vi "Check Axis Faults.vi"(8 "error in (no error)":errorcluster, 11 "Gantry in":refnum<class "Gantry.lvclass">) -> (0 "error out":errorcluster, 3 "Gantry out":refnum<class "Gantry.lvclass">)   [LabVIEW 2026, in "Gantry.lvclass"]
uses:
  Gantry.lvclass
  <instrlib>/Aerotech Automation1/Status/TypeDefs/Axis Fault Cluster.ctl
  <instrlib>/Aerotech Automation1/Status/TypeDefs/Axis Status Items Cluster.ctl
  <instrlib>/Aerotech Automation1/Status/TypeDefs/Axis Status Item.ctl
  <instrlib>/Aerotech Automation1/Status/Wrappers/Add Axis Status Item.vi
  <instrlib>/Aerotech Automation1/Status/Wrappers/Read Axis Status Item.vi
  <instrlib>/Aerotech Automation1/Status/Status.lvlib
  <instrlib>/Aerotech Automation1/Aerotech Automation1.lvlib
panel:
  out "Axis Fault":T1
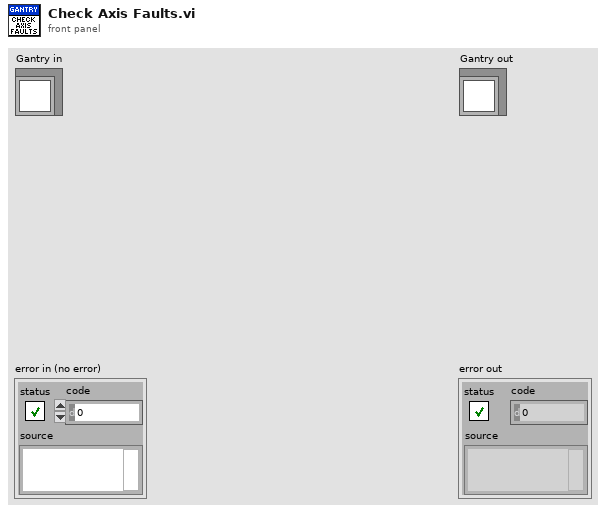
[diagram p1: front panel]
types:
  T1 = typedef "Aerotech Automation1.lvlib/Status.lvlib/Axis Fault Cluster.ctl" = cluster{"PositionErrorFault":bool, "OverCurrentFault":bool, "CwEndOfTravelLimitFault":bool, "CcwEndOfTravelLimitFault":bool, "CwSoftwareLimitFault":bool, "CcwSoftwareLimitFault":bool, "AmplifierFault":bool, "FeedbackInput0Fault":bool, "FeedbackInput1Fault":bool, "HallSensorFault":bool, "MaxVelocityCommandFault":bool, "EmergencyStopFault":bool, "VelocityErrorFault":bool, "Unused 13":bool, "Unused 14":bool, "ExternalFault":bool, "Unused 16":bool, "MotorTemperatureFault":bool, "AmplifierTemperatureFault":bool, "EncoderFault":bool, "Unused 20":bool, "Unused 21":bool, "GantryMisalignmentFault":bool, "FeedbackScalingFault":bool, "MarkerSearchFault":bool, "SafeZoneFault":bool, "InPositionTimeoutFault":bool, "VoltageClampFault":bool, "MotorSupplyFault":bool, "Unused 29":bool, "InternalFault":bool, "Unused 31":bool}
  T2 = typedef "Virtual Modes.ctl" = enum16{"Nonvirtual", "Virtual"}
  T3 = typedef "ControllerDiagPacket.ctl" = cluster{"Number of Diag Packets":i32, "Axes":T4[], "error":errorcluster}
  T4 = typedef "AxisDiagPacket.ctl" = cluster{"Axis Name":string, "Analog Input 0":dbl, "Analog Input 1":dbl, "Axis Fault (num)":i32, "Axis Fault (str)":string, "Axis Fault (bits)":cluster{"AmplifierFault":bool, "AmplifierTemperatureFault":bool, "CcwEndOfTravelLimitFault":bool, "CcwSoftwareLimitFault":bool, "CommunicationLostFault":bool, "CwEndOfTravelLimitFault":bool, "CwSoftwareLimitFault":bool, "EmergencyStopFault":bool, "EncoderFault":bool, "ExternalFault":bool, "FeedbackScalingFault":bool, "GantryMisalignFault ":bool, "HallSensorFault":bool, "InPositionTimeoutFault":bool, "InternalFault":bool, "MarkerSearchFault":bool, "MaxVelocityCommandFault":bool, "MissedInterruptFault":bool, "MotorTemperatureFault":bool, "None":bool, "OverCurrentFault":bool, "PositionErrorFault":bool, "PositionFeedbackFault":bool, "PowerSupplyFault":bool, "ProbeInputFault":bool, "SafeZoneFault":bool, "VelocityErrorFault":bool, "VelocityFeedbackFault":bool, "VoltageClampFault":bool}, "Axis Status (num)":i32, "Axis Status (str)":string, "Axis Status (bits)":cluster{"BacklashActive":bool, "CalibrationEnabled1D":bool, "CalibrationEnabled2D":bool, "CommandValid":bool, "DriveAbortPending":bool, "DrivePending":bool, "Enabling":bool, "GainMappingEnabled":bool, "GantryAligned":bool, "GantryRealigning":bool, "Homed":bool, "Homing":bool, "IFOVEnabled":bool, "JogGenerating":bool, "Jogging":bool, "JoystickControl":bool, "MasterSlaveControl":bool, "MotionBlocked":bool, "MotionClamped":bool, "MoveDone":bool, "None":bool, "NotVirtual":bool, "Profiling":bool, "Stability0":bool, "Stability1":bool, "TrajectoryFiltering":bool, "WaitDone":bool}, "Current Command":sgl, "Current Error":sgl, "Current Feedback":sgl, "Digital Inputs":i32, "Digital Outputs":i32, "Drive Status":i32, "Drive Status (str)":string, "Drive Status (bits)":cluster{"AccelerationPhase":bool, "AutofocusActive":bool, "BrakeOutput":bool, "CcwEndOfTravelLimitInput":bool, "CosineEncoderError":bool, "CurrentClamp":bool, "CwEndOfTravelLimitInput":bool, "DecelerationPhase":bool, "DualLoopActive":bool, "EmergencyStopInput":bool, "Enabled":bool, "EncoderClipping":bool, "GalvoCalibrationEnabled":bool, "GalvoPowerCorrection":bool, "HallAInput":bool, "HallBInput":bool, "HallCInput":bool, "HighResolutionMode":bool, "HomeLimitInput":bool, "InPosition":bool, "InPosition2":bool, "MarkerInput":bool, "MarkerLatch":bool, "MoveActive":bool, "NoMotorSupply":bool, "None":bool, "PowerLimiting":bool, "ProgrammingFlash":bool, "ProgrammingMXH":bool, "PSOHaltLatch":bool, "ServoControl":bool, "SineEncoderError":bool}, "Position Feedback Auxiliary":dbl, "Position Command":dbl, "Position Error":dbl, "Position Feedback":dbl, "Program Position Command":dbl, "Program Position Error":dbl, "Program Position Feedback":dbl, "Velocity Command":dbl, "Velocity Error":dbl, "Velocity Feedback":dbl}
  T5 = typedef "Aerotech Automation1.lvlib/Status.lvlib/Axis Status Items Cluster.ctl" = cluster{"Axis Name":string, "axisStatusItem":T6}
  T6 = typedef "Aerotech Automation1.lvlib/Status.lvlib/Axis Status Item.ctl" = i32
  T7 = typedef "Aerotech Automation1.lvlib/Status.lvlib/Status Refnums.ctl" = cluster{"Status":refnum<k24>, "Status Config":refnum<k24>}
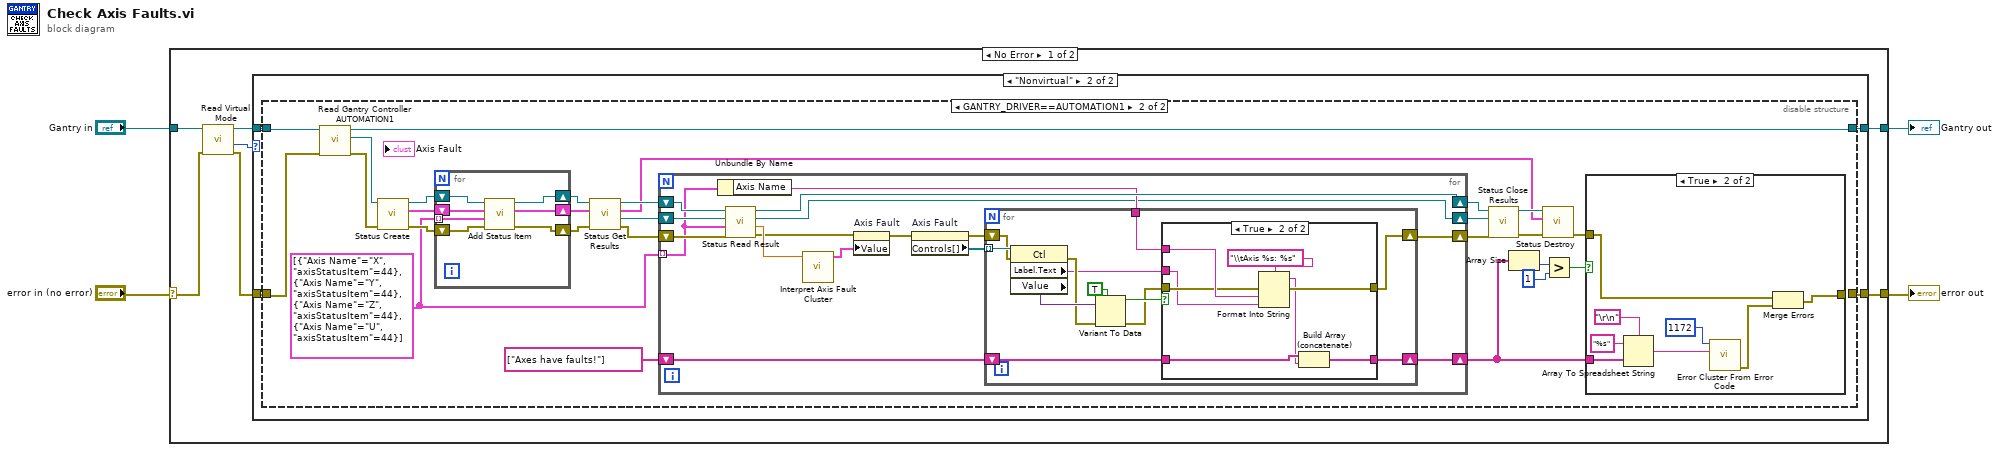
[diagram p0: block diagram]
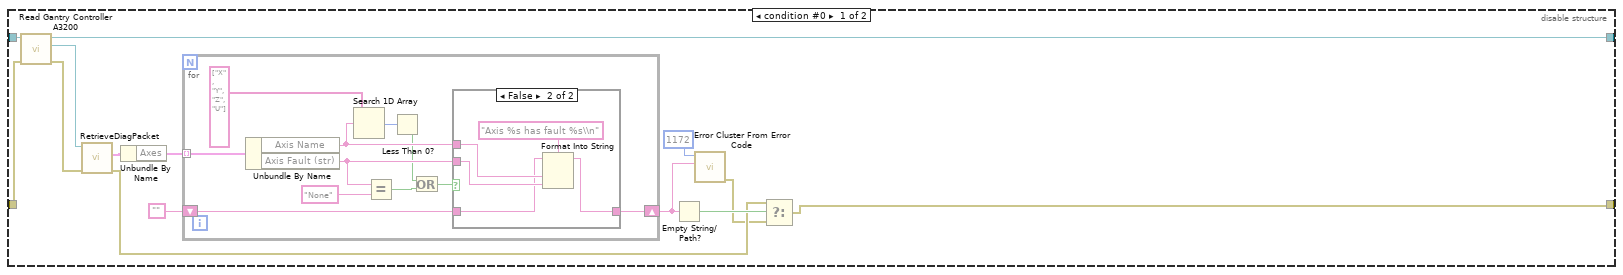
[diagram p3: hidden frame]
diagram:
  n1 = case shown="No Error" "error in (no error)" {
    selector: "error in (no error)" -> [w7 w131]
    tunnel: [w10 w131] -> w3
    tunnel: [w11 w130] -> w1
    tunnel: "Gantry in" -> [w9 w130]
    frame No Error {
      n2 = call-dynamic "Read Virtual Mode.vi"("error in (no error)"=w7, "Gantry in"=w9) -> ("error out"=w6:errorcluster, "Virtual Mode"=w5:T2, "Gantry out"=w8:refnum<class "Gantry.lvclass">)  [unwired: 6 in, 1 out]
      n3 = case shown="\"Nonvirtual\"" w5 {
        tunnel: w6 -> [w12 w14]
        tunnel: w8 -> [w13 w16]
        tunnel: [w13 w15] -> w11
        tunnel: [w12 w17] -> w10
        frame "Virtual" {
        }
        frame "Nonvirtual" {
          n4 = disable-structure shown="GANTRY_DRIVER==AUTOMATION1" {
            disable-tunnel: [w23 _] -> w17
            disable-tunnel: w16 -> [w22 w50]
            disable-tunnel: [w21 w51] -> w15
            disable-tunnel: w14 -> [w20 w49]
            frame condition #0 {
              n5 = call "Read Gantry Controller A3200.vi"("error in (no error)"=w20, "Gantry in"=w22) -> ("error out"=w19:errorcluster, "A3200 controller out"=w18:refnum<k24>, "Gantry out"=w21:refnum<class "Gantry.lvclass">)  [unwired: 7 in]
              n6 = call "RetrieveDiagPacket.vi"("error in (no error)"=w19, "Controller In"=w18) -> ("error out"=w25:errorcluster, "ControllerDiagPacket"=w31:T3)  [unwired: 7 in, 1 out]
              n7 = Unbundle By Name(w31) -> ("Axes"=w30:T4[])
              n8 = for {
                tunnel: w30 -> [w42] mode=indexing
                shift-right: [w38] -> w27
                shift-left: "" -> [w39]
                n9 = Unbundle By Name(w42) -> ("Axis Name"=w36:string, "Axis Fault (str)"=w40:string)
                n10 = Search 1D Array(1D array=string[] ["X", "Y", "Z", "U"], element=w36) -> (index of element=w35:i32)  [unwired: 1 in]
                n11 = Equal?(x=w40, y="None") -> (x = y?=w32:bool)
                n12 = Less Than 0?(x=w35) -> (x < 0?=w34:bool)
                n13 = Or(x=w34, y=w32) -> (x .or. y?=w33:bool)
                n14 = case shown="False" w33 {
                  tunnel: w36 -> [_ w47]
                  tunnel: w40 -> [_ w46]
                  tunnel: w39 -> [w43 w45]
                  tunnel: [w43 w44] -> w38
                  frame True {
                  }
                  frame False {
                    n15 = Format Into String(format string="Axis %s has fault %s\\n", initial string=w45, w47, w46) -> (resulting string=w44:string)  [unwired: 1 in, 1 out]
                  }
                }
              }
              n16 = Empty String/Path?(string/path=w27) -> (empty?=w26:bool)
              n17 = call <vilib>:"Error Cluster From Error Code.vi"("error message (\"\")"=w27, "error code (0)"=1172) -> ("error out"=w24:errorcluster)  [unwired: 7 in]
              n18 = Select(t=w25, s=w26, f=w24) -> (s? t:f=w23:errorcluster)
            }
            frame condition #1 (active) {
              w60 = T5[] [{"Axis Name"="X", "axisStatusItem"=44}, {"Axis Name"="Y", "axisStatusItem"=44}, {"Axis Name"="Z", "axisStatusItem"=44}, {"Axis Name"="U", "axisStatusItem"=44}]
              n19 = call "Read Gantry Controller AUTOMATION1.vi"("error in (no error)"=w49, "Gantry in"=w50) -> ("error out"=w74:errorcluster, "Controller AUTOMATION1"=w75:refnum<k24>, "Gantry out"=w51:refnum<class "Gantry.lvclass">)  [unwired: 7 in]
              n20 = call <instrlib>:"Status Create.vi"("error in (no error)"=w74, "Controller Refnum"=w75) -> ("error out"=w72:errorcluster, "Status Refnums"=w73:T7, "Controller Refnum out"=w71:refnum<k24>)  [unwired: 7 in]
              n21 = for {
                tunnel: w60 -> [w126] mode=indexing
                shift-right: [w125] -> w68
                shift-left: w73 -> [w129]
                shift-right: [w124] -> w70
                shift-left: w71 -> [w127]
                shift-right: [w123] -> w69
                shift-left: w72 -> [w128]
                n22 = call-poly <instrlib>:"Add Status Item.vi"("error in"=w128, "Axis Status Item"=w126, "Status Refnums"=w129, "Controller Refnum"=w127) -> ("error out"=w123:errorcluster, "Status Refnums out"=w125:T7, "Controller Refnum out"=w124:refnum<k24>)  [unwired: 5 in]
              }
              n23 = call <instrlib>:"Status Get Results.vi"("error in (no error)"=w69, "Status Refnums"=w68, "Controller Refnum"=w70) -> ("error out"=w66:errorcluster, "GetStatusItems"=w65:refnum<k24>, "Status Refnums out"=w59:T7, "Controller Refnum out"=w67:refnum<k24>)  [unwired: 5 in]
              n24 = for {
                shift-right: [w96] -> w62
                shift-left: w67 -> [w99]
                shift-right: [w86] -> w58
                shift-left: w66 -> [w98]
                tunnel: w60 -> [w90] mode=indexing
                shift-right: [w88] -> w52
                shift-left: string[] ["Axes have faults!"] -> [w89]
                shift-right: [w85] -> w63
                shift-left: w65 -> [w100]
                n25 = Unbundle By Name(w90) -> ("Axis Name"=w87:string)
                n26 = call-poly <instrlib>:"Status Read Result.vi"("error in (no error)"=w98, "Axis Status Item"=w90, "Status Results Refnum"=w100, "Controller Refnum"=w99) -> ("error out"=w94:errorcluster, "Data"=w97:dbl, "Status Results Refnum out"=w85:refnum<k24>, "Controller Refnum out"=w96:refnum<k24>)  [unwired: 4 in]
                n27 = call <instrlib>:"Interpret Axis Fault Cluster.vi"("Data"=w97) -> ("Axis Fault Cluster"=w95:T1)  [unwired: 10 in]
                n28 = property on="Axis Fault" class="Clust (strict)"(error in=w94, "Value"=w95) -> (error out=w93:errorcluster)  [unwired: 1 in, 1 out]
                n29 = property on="Axis Fault" class="Clust (strict)"(error in=w93) -> (error out=w91:errorcluster, "Controls[]"=w92:refnum<vi>[])  [unwired: 1 in, 1 out]
                n30 = for {
                  tunnel: w92 -> [w112] mode=indexing
                  shift-right: [w105] -> w88
                  shift-left: w89 -> [w106]
                  shift-right: [w101] -> w86
                  shift-left: w91 -> [w109]
                  tunnel: w87 -> [w103]
                  n31 = property class="Ctl"(reference=w112, error in=w109) -> (error out=w108:errorcluster, "Label.Text"=w104:string, "Value"=w111:variant)  [unwired: 1 out]
                  n32 = Variant To Data(error in=w108, type=TRUE, Variant=w111) -> (data=w107:bool, error out=w102:errorcluster)
                  n33 = case shown="True" w107 {
                    tunnel: w106 -> [w114 w117]
                    tunnel: [w114 w116] -> w105
                    tunnel: w104 -> [_ w118]
                    tunnel: w103 -> [_ w121]
                    tunnel: w102 -> [w113 w120]
                    tunnel: [w113 w119] -> w101
                    frame False {
                    }
                    frame True {
                      n34 = Format Into String(format string="\\tAxis %s: %s", error in=w120, w121, w118) -> (resulting string=w115:string, error out=w119:errorcluster)  [unwired: 1 in]
                      n35 = Build Array (concatenate)(w117, w115) -> (w116:string[])
                    }
                  }
                }
              }
              n36 = call <instrlib>:"Status Close Results.vi"("error in (no error)"=w58, "Status Results Refnum"=w63, "Controller Refnum"=w62) -> ("error out"=w57:errorcluster, "Controller Refnum out"=w61:refnum<k24>)  [unwired: 7 in]
              n37 = Array Size(array=w52) -> (size(s)=w54:i32)
              n38 = call <instrlib>:"Status Destroy.vi"("error in"=w57, "Status Refnums"=w59, "Controller Refnum"=w61) -> ("error out"=w56:errorcluster)  [unwired: 7 in, 1 out]
              n39 = Greater?(x=w54, y=1) -> (0:w55:bool)
              n40 = case shown="True" w55 {
                tunnel: w56 -> [w76 w80]
                tunnel: w52 -> [_ w84]
                tunnel: [w76 w78] -> _
                frame False {
                }
                frame True {
                  n41 = Array To Spreadsheet String(delimiter (Tab)="\r\n", array=w84, 3:"%s" ("format string")) -> (spreadsheet string=w82:string)
                  n42 = call <vilib>:"Error Cluster From Error Code.vi"("error message (\"\")"=w82, "error code (0)"=1172) -> ("error out"=w79:errorcluster)  [unwired: 7 in]
                  n43 = Merge Errors(w80, w79) -> (w78:errorcluster)
                }
              }
            }
          }
        }
      }
    }
    frame Error {
    }
  }
  "error out" <- w3
  "Gantry out" <- w1
